vi "Start Test.vi"(8 "error in (no error)":errorcluster, 10 "Tests":string[](array[string]), 11 "Result Model In":refnum<class "Result Model.lvclass">) -> (0 "error out":errorcluster, 3 "Result Model Out":refnum<class "Result Model.lvclass">)   [LabVIEW 2020, in "Result Model.lvclass"]
uses:
  Result Model.lvclass
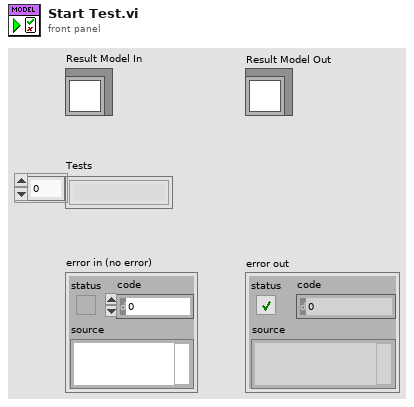
[diagram p1: front panel]
types:
  T1 = typedef "Result.lvlib/Status.ctl" = enum16{"", "Passed", "Failed", "Error", "Skipped", "Setup Error", "Broken", "Teardown Error"}
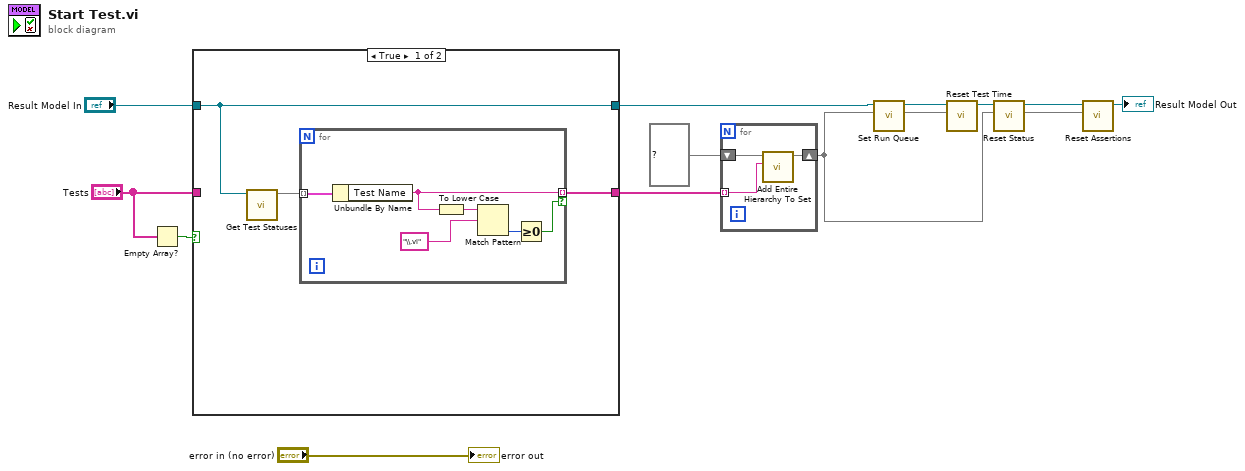
[diagram p0: block diagram]
diagram:
  n1 = Empty Array?(array="Tests") -> (empty?=w11:bool)
  n2 = case shown="True" w11 {
    tunnel: "Result Model In" -> [w14 w23]
    tunnel: [w14 w23] -> w7
    tunnel: "Tests" -> [_ w22]
    tunnel: [w13 w22] -> w8
    frame True {
      n3 = call "Get Test Statuses.vi"("Result Model In"=w14) -> ("Test Statuses"=w15:map{string, T1})  [unwired: 10 in]
      n4 = for {
        tunnel: w15 -> [w21] mode=indexing
        tunnel: [w17] -> w13 mode=indexing if=w16
        n5 = Unbundle By Name(w21) -> ("Test Name"=w17:string)
        n6 = To Lower Case(string=w17) -> (all lower case string=w18:string)
        n7 = Match Pattern(string=w18, regular expression="\\.vi") -> (offset past match=w19:i32)  [unwired: 1 in, 3 out]
        n8 = Greater Or Equal To 0?(x=w19) -> (x >= 0?=w16:bool)
      }
    }
    frame False {
    }
  }
  n9 = for {
    shift-right: [w25] -> w6
    shift-left: set{string} {} ("Run Queue") -> [w26]
    tunnel: w8 -> [w24] mode=indexing
    n10 = call "Add Entire Hierarchy To Set.vi"("Test Name"=w24, "Set in"=w26) -> ("Set out"=w25:set{string})  [unwired: 9 in]
  }
  n11 = call "Set Run Queue.vi"("Run Queue"=w6, "Result Model In"=w7) -> ("Result Model Out"=w2:refnum<class "Result Model.lvclass">)  [unwired: 9 in]
  n12 = call "Reset Test Time.vi"("Run Queue"=w6, "Result Model In"=w2) -> ("Result Model Out"=w3:refnum<class "Result Model.lvclass">)  [unwired: 9 in]
  n13 = call "Reset Status.vi"("Run Queue"=w6, "Result Model In"=w3) -> ("Result Model Out"=w4:refnum<class "Result Model.lvclass">)  [unwired: 9 in]
  n14 = call "Reset Assertions.vi"("Run Queue"=w6, "Result Model In"=w4) -> ("Result Model Out"=→"Result Model Out":refnum<class "Result Model.lvclass">)  [unwired: 9 in]
  "error out" <- "error in (no error)"
